vi "DO Configuration to Channel Settings.vi"(8 "error in":errorcluster, 9 "default values":dbl[](array[numeric]), 10 "names":string[](array[string]), 11 "mode in":refnum<class "Mode.lvclass">) -> (0 "error out":errorcluster, 2 "channel settings":T1[](array[typedef]), 3 "mode out":refnum<class "Mode.lvclass">)   [LabVIEW 2017, in "Scan Engine Scripting.lvlib" / "Mode.lvclass"]
uses:
  Mode.lvclass
  Controls/digital channel settings.ctl
  Scan Engine Scripting.lvlib
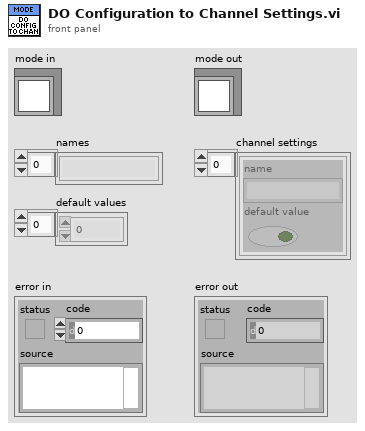
[diagram p1: front panel]
types:
  T1 = typedef "Scan Engine Scripting.lvlib/digital channel settings.ctl" = cluster{"name":string, "default value":bool}
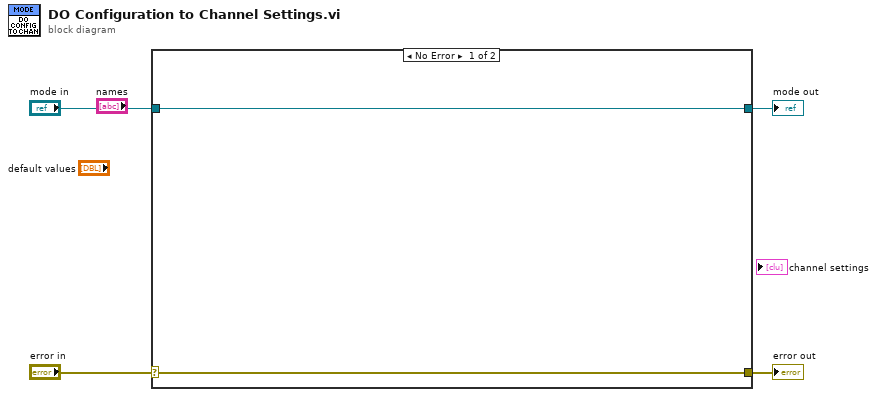
[diagram p0: block diagram]
diagram:
  n1 = case shown="No Error" "error in" {
    selector: "error in" -> [w5 w8]
    tunnel: [w5 w8] -> w3
    tunnel: [w6 w7] -> w1
    tunnel: "mode in" -> [w6 w7]
    frame No Error {
    }
    frame Error {
    }
  }
  "error out" <- w3
  "mode out" <- w1
